vi "readFromXML.vi"(8 "error in (no error)":errorcluster, 10 "XML in":string, 11 "WavefrontTargetClearOffset in":refnum<class "WavefrontTargetClearOffset.lvclass">) -> (0 "error out":errorcluster, 3 "WavefrontTargetClearOffset out":refnum<class "WavefrontTargetClearOffset.lvclass">)   [LabVIEW 2022 SP3, in "TCSDataDefinitions.lvlib" / "TCSCommand.lvlib" / "OffsetCommands.lvlib" / "WavefrontTargetClearOffset.lvclass"]
uses:
  WavefrontTargetClearOffset.lvclass
  ClearOffset/ClearOffset.lvclass
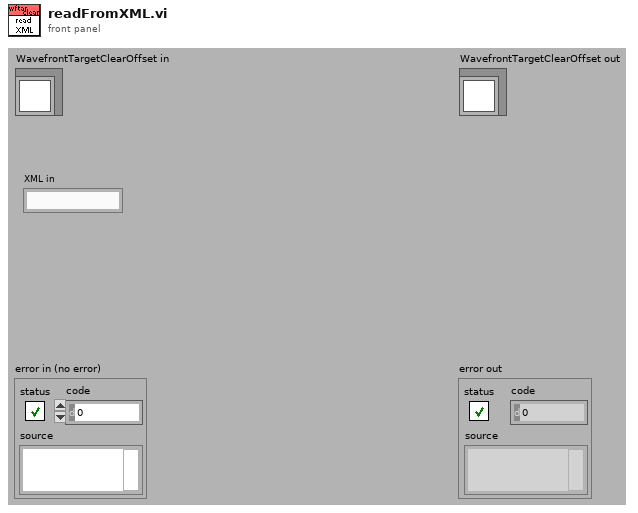
[diagram p1: front panel]
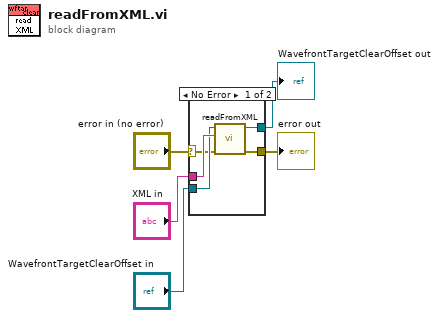
[diagram p0: block diagram]
diagram:
  n1 = case shown="No Error" "error in (no error)" {
    selector: "error in (no error)" -> [w6 w12]
    tunnel: [w10 w12] -> w5
    tunnel: [w9 w11] -> w4
    tunnel: "XML in" -> [w8 _]
    tunnel: "WavefrontTargetClearOffset in" -> [w7 w11]
    frame No Error {
      n2 = call-parent "readFromXML.vi"("error in (no error)"=w6, "XML in"=w8, "ClearOffset in"=w7) -> ("error out"=w10:errorcluster, "ClearOffset out"=w9:refnum<class "WavefrontTargetClearOffset.lvclass">)  [unwired: 7 out]
    }
    frame Error {
    }
  }
  "error out" <- w5
  "WavefrontTargetClearOffset out" <- w4
